vi "WriteIO.fifodirect.fpga.vi"(9 "Delta time":i32, 10 "Number of time points":i32) -> ()   [LabVIEW 2012]
uses:
  <vilib>/rvi/interface/RandomDataEmulation/nirviRandomDataFPGAFIFO.vi
  <vilib>/rvi/interface/RandomDataEmulation/niFpgaRandomDataHandleErrors.vi
  <vilib>/rvi/DataTransferAndStorage/Container/XNode/niFpgaContainer.xnode
  <vilib>/rvi/interface/RandomDataEmulation/nirviRandomDataFpgaReadWriteTemplate.vi
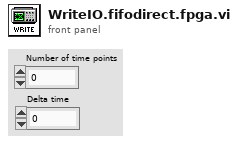
[diagram p1: front panel]
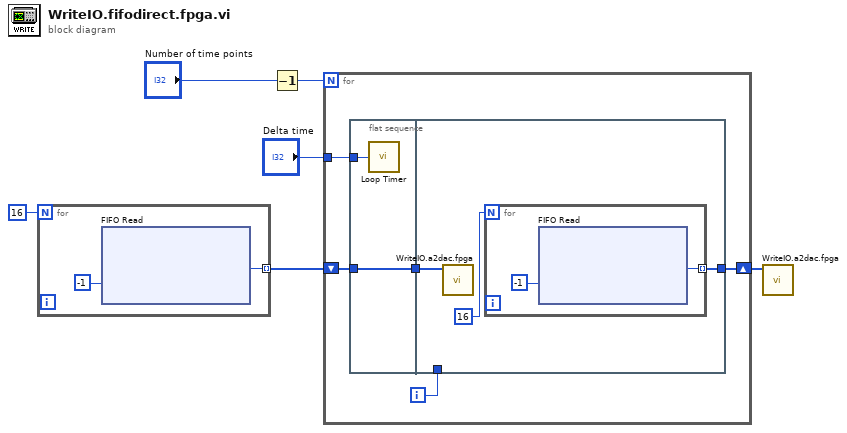
[diagram p0: block diagram]
diagram:
  n1 = for {
    N: 16 -> [_]
    tunnel: [w8] -> w4 mode=indexing
    n2 = xnode "FIFO Read"("Timeout"=-1) -> ("Element"=w8:i16)  [unwired: 1 in, 2 out]
  }
  n3 = Decrement(x="Number of time points") -> (x-1=w1:i32)
  n4 = for {
    N: w1 -> [_]
    tunnel: "Delta time" -> [w13]
    shift-right: [w9] -> w3
    shift-left: w4 -> [w10]
    i -> [w12]
    n5 = flat-sequence {
      tunnel: w13 -> [w15]
      tunnel: [w14] -> w11
      tunnel: w10 -> [w14]
      tunnel: w12 -> [_]
      tunnel: w11 -> [w17]
      tunnel: [w16] -> w9
      frame #0 {
        n6 = call "Loop Timer"("Count(Ticks)"=w15) -> ()  [unwired: 1 out]
      }
      frame #1 {
        n7 = call "WriteIO.a2dac.fpga.vi"("Array"=w17) -> ()  [unwired: 11 in]
        n8 = for {
          N: 16 -> [_]
          tunnel: [w20] -> w16 mode=indexing
          n9 = xnode "FIFO Read"("Timeout"=-1) -> ("Element"=w20:i16)  [unwired: 1 in, 2 out]
        }
      }
    }
  }
  n10 = call "WriteIO.a2dac.fpga.vi"("Array"=w3) -> ()  [unwired: 11 in]
